vi "Available VISA Resources.vi"() -> ()   [LabVIEW 2012]
doc: "SciScan 1.2 160622"
panel:
  out "Interface Type":string[][](array[string])
  out "Resource Names":string[](array[string])
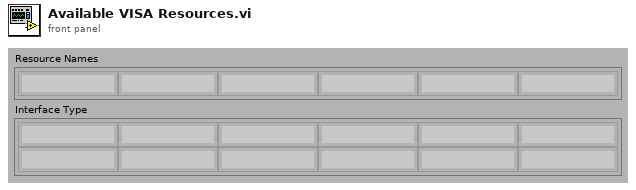
[diagram p1: front panel]
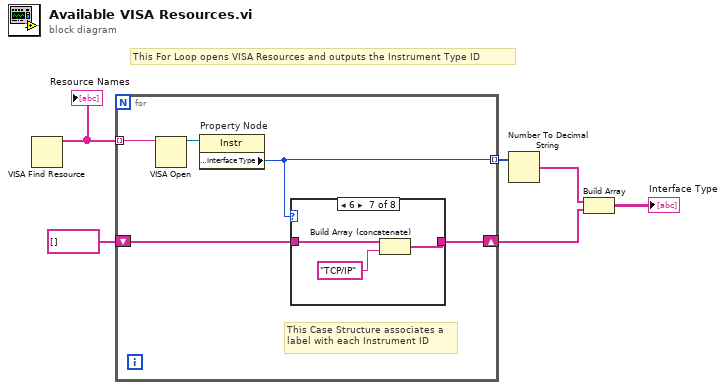
[diagram p0: block diagram]
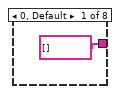
[diagram p2: hidden frame]
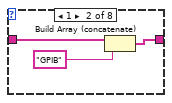
[diagram p3: hidden frame]
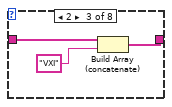
[diagram p4: hidden frame]
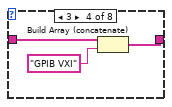
[diagram p5: hidden frame]
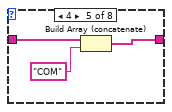
[diagram p6: hidden frame]
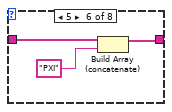
[diagram p7: hidden frame]
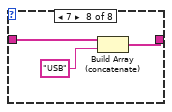
[diagram p8: hidden frame]
diagram:
  # "This For Loop opens VISA Resources and outputs the Instrument Type ID"
  n1 = VISA Find Resource() -> (3:w2:string[])  [unwired: 3 in, 2 out]
  "Resource Names" <- w2
  n2 = for {
    tunnel: w2 -> [w11] mode=indexing
    tunnel: [w8] -> w5 mode=indexing
    shift-right: [w10] -> w3
    shift-left: string[] [] -> [w9]
    # "This Case Structure associates a \nlabel with each Instrument ID"
    n3 = VISA Open(VISA resource name=w11) -> (VISA resource name=w7:refnum<visa-resource-name>)  [unwired: 4 in, 1 out]
    n4 = property on="Property Node" class="Instr"(reference=w7) -> ("Interface Information:Interface Type"=w8:u16)  [unwired: 1 in, 2 out]
    n5 = case shown="6" w8 {
      tunnel: [string[] [] w14 w18 w21 w22 w27 w30 w33] -> w10
      tunnel: w9 -> [_ w13 w16 w20 w24 w26 w29 w32]
      frame 0, Default {
      }
      frame 1 {
        n6 = Build Array (concatenate)(w13, "GPIB") -> (w14:string[])
      }
      frame 2 {
        n7 = Build Array (concatenate)(w16, "VXI") -> (w18:string[])
      }
      frame 3 {
        n8 = Build Array (concatenate)(w20, "GPIB VXI") -> (w21:string[])
      }
      frame 4 {
        n9 = Build Array (concatenate)(w24, "COM") -> (w22:string[])
      }
      frame 5 {
        n10 = Build Array (concatenate)(w26, "PXI") -> (w27:string[])
      }
      frame 6 {
        n11 = Build Array (concatenate)(w29, "TCP/IP") -> (w30:string[])
      }
      frame 7 {
        n12 = Build Array (concatenate)(w32, "USB") -> (w33:string[])
      }
    }
  }
  n13 = Number To Decimal String(number=w5) -> (decimal integer string=w4:string[])  [unwired: 1 in]
  n14 = Build Array "Build Array"(w4, w3) -> (→"Interface Type":string[][])
